vi "UnPark_from_EoL.vi"(3 "offset Y":dbl, 4 "offset X":dbl, 5 "Line_start":i32, 6 "Range":dbl=10.0, 7 "Pixels":i32=256, 8 "dwell":dbl=1.0) -> (0 "X and Y":waveform(dbl)[](array[waveform]), 1 "Array Y":dbl[](array[numeric]), 2 "Array X":dbl[](array[numeric]))   [LabVIEW 2016]
panel:
  out "size(s)":i32
  out "start line Y":dbl
  out "Waveform Graph":waveform(dbl)[](graph)
  out "start line X":dbl
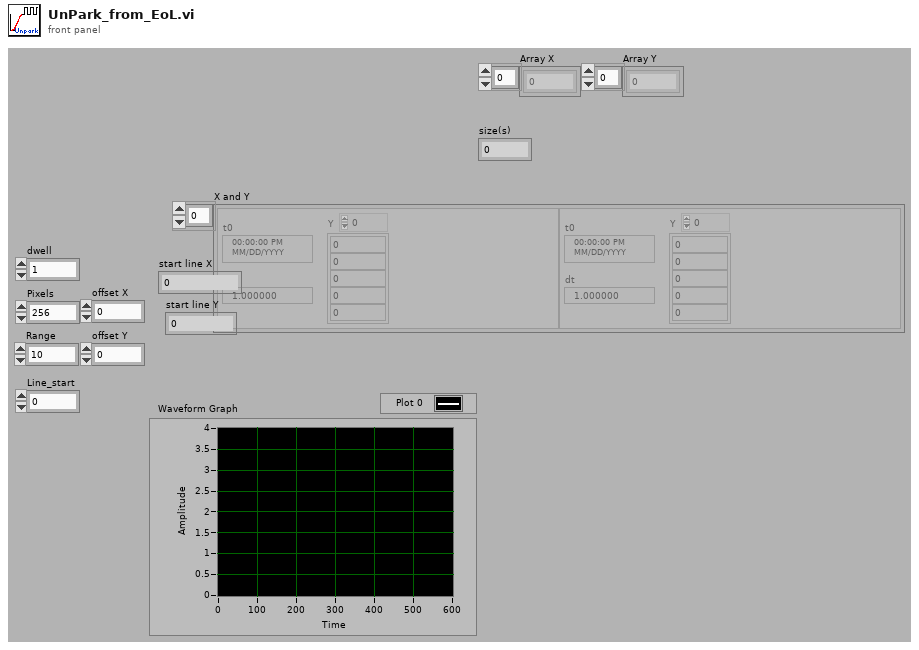
[diagram p1: front panel]
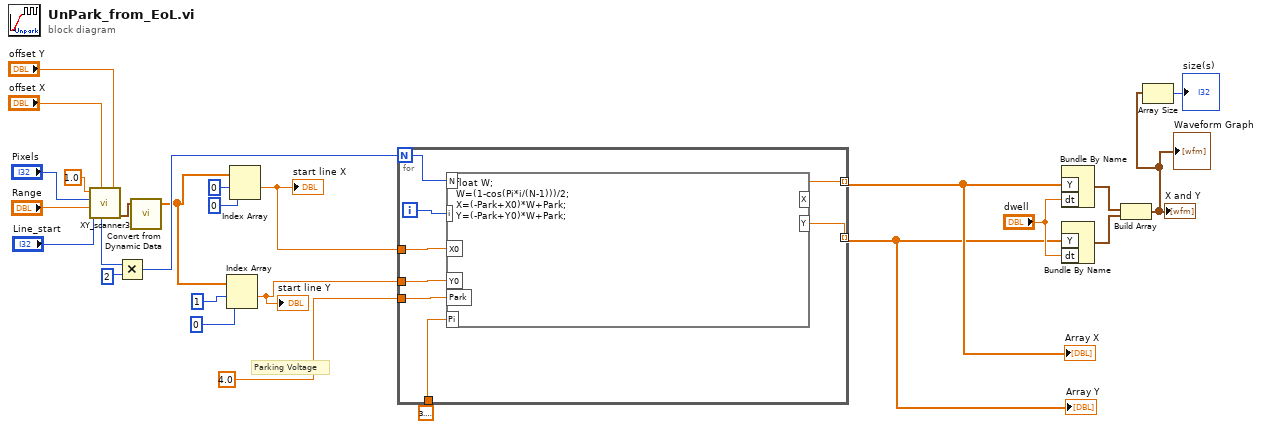
[diagram p0: block diagram]
diagram:
  # "Parking Voltage"
  n1 = call "XY_scanner3.vi"("offset Y"="offset Y", "offset X"="offset X", "Line_start"="Line_start", "Range"="Range", "Pixels"="Pixels", "dwell"=1.0) -> ("X and Y"=w1:waveform(dbl)[], "scanPix"=w17:i32)  [unwired: 2 out]
  n2 = Multiply(x=w17, y=2) -> (x*y=w16:i32)
  n3 = call "Convert from Dynamic Data"("Dynamic Data Type"=w1) -> ("Array"=w8:dbl[])  [unwired: 3 in]
  n4 = Index Array(array=w8, index #1=1 ("index"), index #2=0 ("index")) -> (element #1=w7:dbl)  [unwired: 1 out]
  "start line Y" <- w7
  n5 = Index Array(array=w8, index #1=0 ("index"), index #2=0 ("index")) -> (element #1=w11:dbl)  [unwired: 1 out]
  "start line X" <- w11
  n6 = for {
    N: w16 -> [w33]
    tunnel: 3.141592653589793 -> [w32]
    tunnel: [w31] -> w5 mode=indexing
    tunnel: [w30] -> w4 mode=indexing
    tunnel: w11 -> [w29]
    tunnel: w7 -> [w28]
    tunnel: 4.0 ("input variable") -> [w27]
    i -> [w34]
    n7 = formula code="float W;\nW=(1-cos(Pi*i/(N-1)))/2;\nX=(-Park+X0)*W+Park;\nY=(-Park+Y0)*W+Park;"("N"=w33, "i"=w34, "Pi"=w32, "X0"=w29, "Y0"=w28, "Park"=w27) -> ("X"=w31:dbl, "Y"=w30:dbl)
  }
  "Array X" <- w5
  "Array Y" <- w4
  n8 = Bundle By Name("Y"=w5, "dt"="dwell") -> (w21:waveform(dbl))  [unwired: 1 in]
  n9 = Bundle By Name("Y"=w4, "dt"="dwell") -> (w20:waveform(dbl))  [unwired: 1 in]
  n10 = Build Array(w21, w20) -> (w3:waveform(dbl)[])
  "X and Y" <- w3
  "Waveform Graph" <- w3
  n11 = Array Size(array=w3) -> (size(s)=→"size(s)":i32)
